vi "Run.vi"(8 "error in (no error)":errorcluster caption="entrée d'erreur (pas d'erreur)", 11 "lfw_pairs.lvclass":refnum<class "lfw_pairs.lvclass">) -> (0 "error out":errorcluster caption="sortie d'erreur", 2 "Data":T1, 3 "lfw_pairs.lvclass":refnum<class "lfw_pairs.lvclass">)   [LabVIEW 2020, in "lfw_pairs.lvclass"]
doc: "Returns :\n\n- data : ndarray of shape (2200, 2, 62, 47). Shape depends on subset\nEach row has 2 face images corresponding to same or different person from the dataset containing 5749 people. Changing the slice_, resize or subset parameters will change the shape of the output.\n\n- target : numpy array of shape (2200,). Shape depends on subset.\nLabels associated to each pair of images. The two label values being different persons or the same person."
uses:
  lfw_pairs.lvclass
  lfw_pairs.lvclass/lfw_pairs.ctl
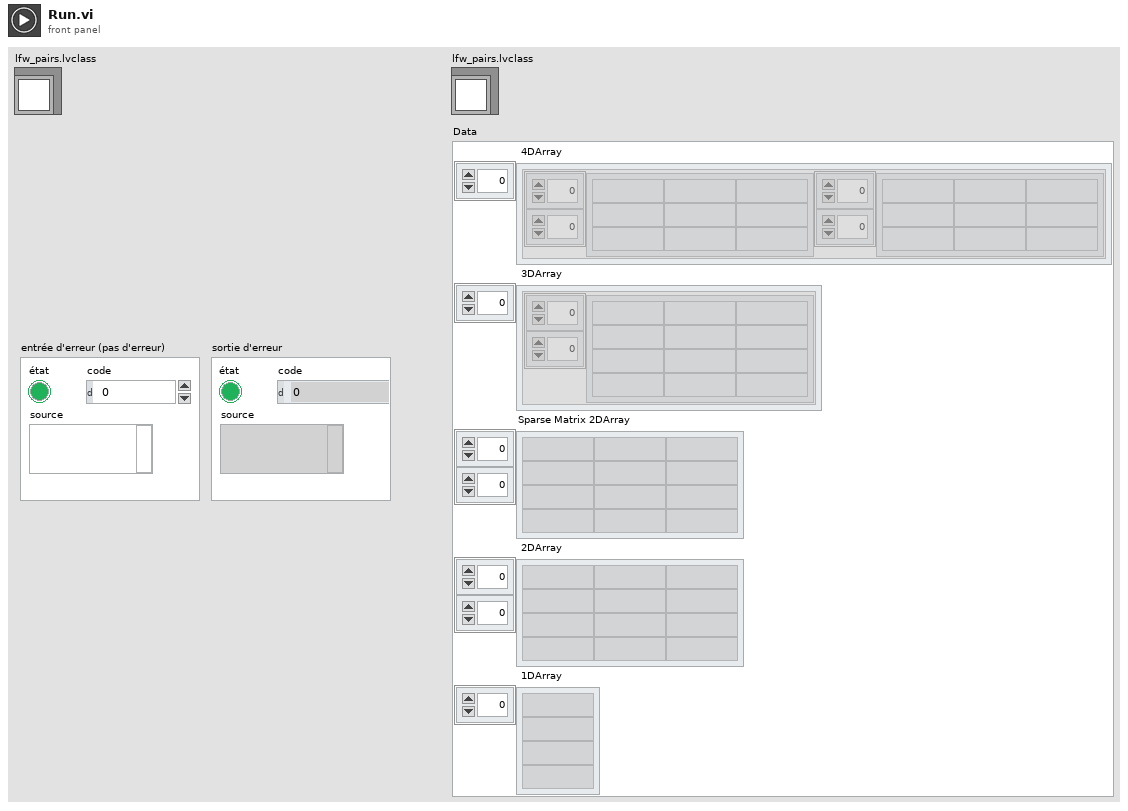
[diagram p1: front panel]
types:
  T1 = cluster{" 4DArray":cluster{"1":string[][], "2":string[][]}[], " 3DArray":cluster{"Tableau":string[][]}[], "Sparse Matrix 2DArray":string[][], " 2DArray":string[][], " 1DArray":string[]}
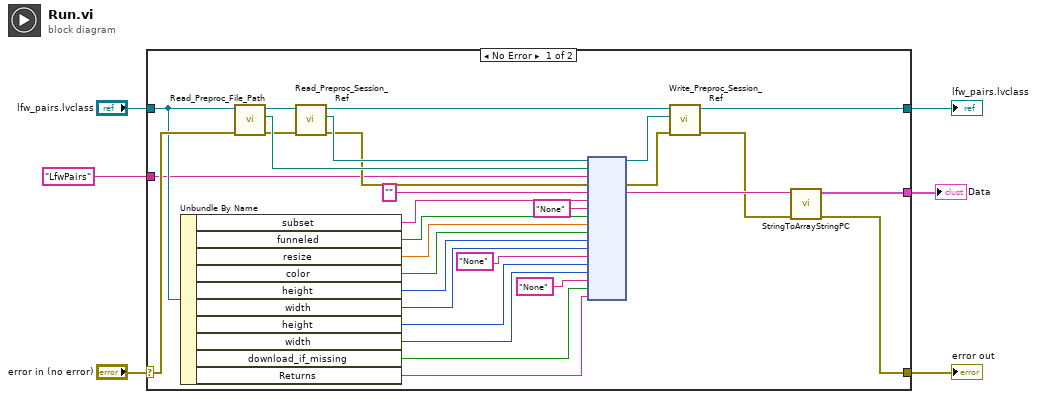
[diagram p0: block diagram]
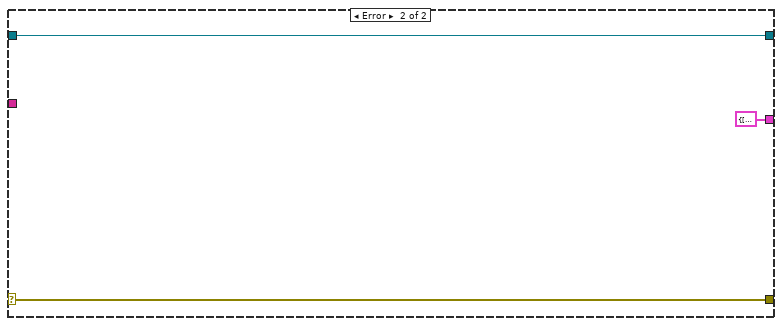
[diagram p2: hidden frame]
diagram:
  n1 = case shown="No Error" "error in (no error)" {
    selector: "error in (no error)" -> [w28 w39]
    tunnel: [w8 w39] -> w5
    tunnel: [w11 w38] -> w3
    tunnel: "lfw_pairs.lvclass" -> [w27 w38]
    tunnel: "LfwPairs" -> [w26 _]
    tunnel: [w7 T1 {" 4DArray"=[], " 3DArray"=[], "Sparse Matrix 2DArray"=[], " 2DArray"=[], " 1DArray"=[]} ("Data")] -> w1
    frame No Error {
      n2 = Unbundle By Name(w27) -> ("subset"=w15:string, "funneled"=w25:bool, "resize"=w24:dbl, "color"=w23:bool, "height"=w22:u32, "width"=w21:u32, "height"=w19:u32, "width"=w18:u32, "download_if_missing"=w16:bool, "Returns"=w12:string)
      n3 = call-dynamic "Read_Preproc_File_Path.vi"("error in (no error)"=w28, "Python in"=w27) -> ("error out"=w31:errorcluster, "File_Path"=w34:path, "Python out"=w36:refnum<class "lfw_pairs.lvclass">)  [unwired: 7 in]
      n4 = call-dynamic "Read_Preproc_Session_Ref.vi"("error in (no error)"=w31, "Python in"=w36) -> ("error out"=w32:errorcluster, "Session_ref"=w33:refnum<k35>, "Python out"=w35:refnum<class "lfw_pairs.lvclass">)  [unwired: 7 in]
      n5 = node(w33, w34, w26, w32, "", w15, "None", w25, w24, w23, w22, w21, "None", w19, w18, "None", w16, w12) -> (w29:refnum<k35>, w13:errorcluster, w10:string)  [unwired: 13 in, 2 out]
      n6 = call-dynamic "Write_Preproc_Session_Ref.vi"("error in (no error)"=w13, "Session_ref"=w29, "Python in"=w35) -> ("error out"=w9:errorcluster, "Python out"=w11:refnum<class "lfw_pairs.lvclass">)  [unwired: 7 in]
      n7 = call "StringToArrayStringPC.vi"("sortie d'erreur"=w9, "Return value"=w10) -> ("sortie d'erreur"=w8:errorcluster, "Data"=w7:T1)  [unwired: 8 in]
    }
    frame Error {
    }
  }
  "error out" <- w5
  "lfw_pairs.lvclass" <- w3
  "Data" <- w1
